vi "Init.vi"(8 "error in (no error)":errorcluster, 11 "Thermometer DAQmx Config in":refnum<class "Thermometer DAQmx Config.lvclass">) -> (0 "error out":errorcluster, 3 "Thermometer DAQmx Config out":refnum<class "Thermometer DAQmx Config.lvclass">)   [LabVIEW 2023, in "Thermometer.lvlib" / "Thermometer DAQmx.lvlib" / "Thermometer DAQmx Config.lvclass"]
uses:
  Thermometer DAQmx Config.lvclass
  Thermometer DAQmx Config.lvclass/Thermometer DAQmx Config.ctl
  Configuration Base/Configuration Base.lvclass
  62684682-e575-4010-bfc8-5be8010980ed.vi
  <vilib>/Utility/error.llb/Error Cluster From Error Code.vi
  <vilib>/ErrorRing/Error Ring.xnode
  D:/git/HAL/Configuration Base/Configuration Base.lvclass
  D:/git/HAL/Interfaces/IConfigure IAI/IConfigure IAI.lvclass
  D:/git/HAL/Interfaces/IConfigure/IConfigure.lvclass
  D:/git/HAL/Interfaces/IConfigure Thermometer/IConfigure Thermometer.lvclass
  D:/git/HAL/Thermometer/Thermometer DAQmx/Thermometer DAQmx Config/Thermometer DAQmx Config.lvclass
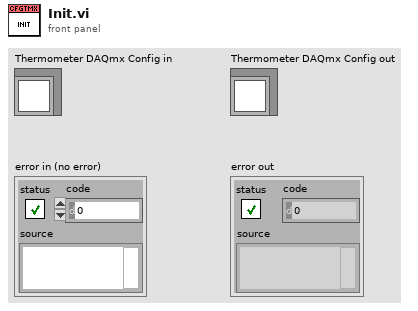
[diagram p1: front panel]
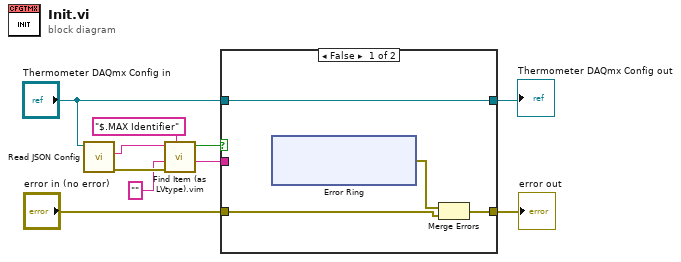
[diagram p0: block diagram]
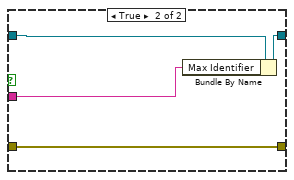
[diagram p2: hidden frame]
diagram:
  n1 = call "Read JSON Config.vi"("object in"="Thermometer DAQmx Config in") -> ("error out"=w9:errorcluster, "<JSON>Config"=w10:string)  [unwired: 8 in, 1 out]
  n2 = call "Find Item (as LVtype).vim"("$Path or Item Name"="$.MAX Identifier", "error in (no error)"=w9, "Data Type and Default Value"="", "JSON"=w10) -> ("Data"=w6:string, "Found"=w2:bool)  [unwired: 4 in, 2 out]
  n3 = case shown="False" w2 {
    tunnel: "error in (no error)" -> [w12 w23]
    tunnel: [w14 w23] -> w5
    tunnel: [w11 w22] -> w3
    tunnel: "Thermometer DAQmx Config in" -> [w11 w21]
    tunnel: w6 -> [_ w20]
    frame False {
      n4 = xnode "Error Ring"() -> ("error out"=w13:errorcluster)
      n5 = Merge Errors(w13, w12) -> (w14:errorcluster)
    }
    frame True {
      n6 = Bundle By Name(cluster=w21, "Max Identifier"=w20) -> (w22:refnum<class "Thermometer DAQmx Config.lvclass">)
    }
  }
  "error out" <- w5
  "Thermometer DAQmx Config out" <- w3
